vi "Cycle Begin.vi"(8 "error in (no error)":errorcluster, 11 "Performance in":refnum<class "Performance.lvclass">) -> (0 "error out":errorcluster, 3 "Performance out":refnum<class "Performance.lvclass">)   [LabVIEW 2019, in "DSF Core.lvlib" / "Performance.lvclass"]
uses:
  Performance.lvclass
  Performance.lvclass/Performance.ctl
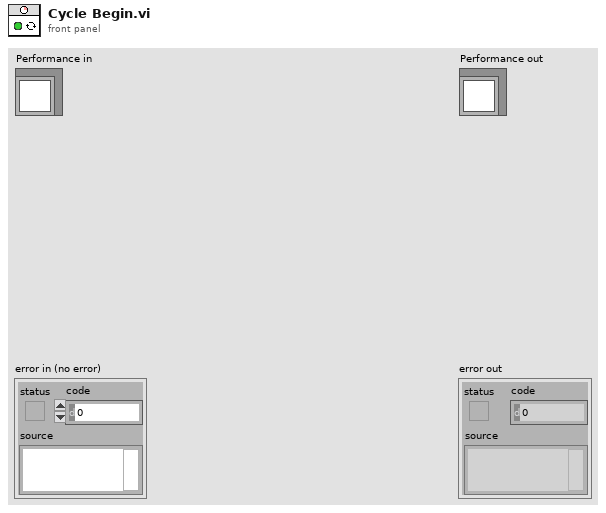
[diagram p1: front panel]
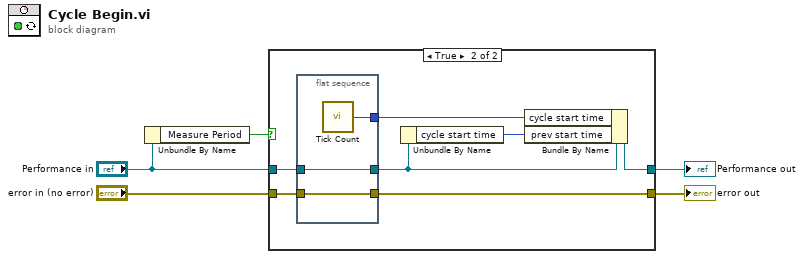
[diagram p0: block diagram]
diagram:
  n1 = Unbundle By Name("Performance in") -> ("Measure Period"=w1:bool)
  n2 = case shown="True" w1 {
    tunnel: [w6 w12] -> w5
    tunnel: "error in (no error)" -> [w6 w14]
    tunnel: [w7 w11] -> w3
    tunnel: "Performance in" -> [w7 w13]
    frame False {
    }
    frame True {
      n3 = flat-sequence {
        tunnel: w13 -> [w17]
        tunnel: w14 -> [w16]
        tunnel: [w17] -> w9
        tunnel: [w16] -> w12
        tunnel: [w15] -> w10
        frame #0 {
          n4 = call "Tick Count"() -> ("Tick Count(uSec)"=w15:u32)
        }
      }
      n5 = Unbundle By Name(w9) -> ("cycle start time"=w8:u32)
      n6 = Bundle By Name(cluster=w9, "cycle start time"=w10, "prev start time"=w8) -> (w11:refnum<class "Performance.lvclass">)
    }
  }
  "error out" <- w5
  "Performance out" <- w3
